vi "sposta nuove colonne.vi"(11 "Array 5":string[][](array[string])) -> (3 "Array 4":string[][](array[string]))   [LabVIEW 2019]
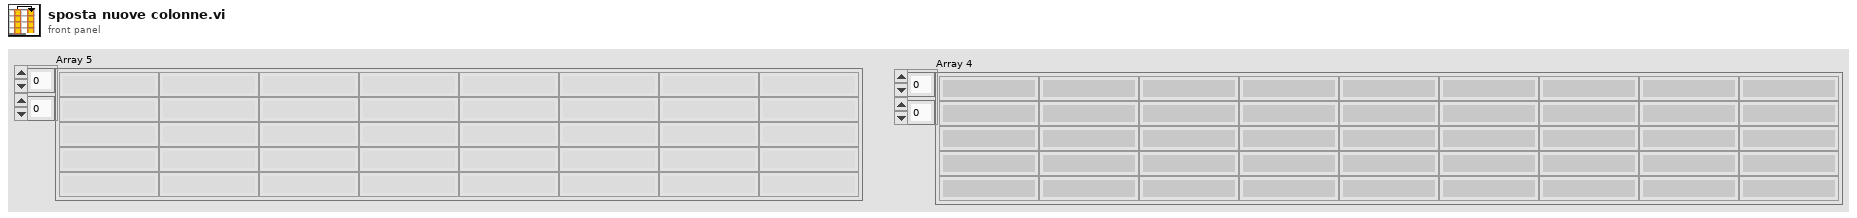
[diagram p1: front panel]
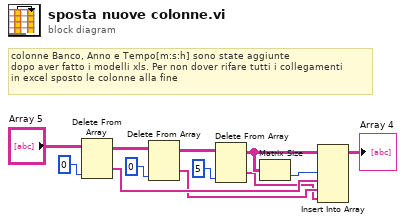
[diagram p0: block diagram]
diagram:
  # "colonne Banco, Anno e Tempo[m:s:h] sono state aggiunte\ndopo aver fatto i modelli xls. Per non dover rifare tutti i collegamenti\nin excel sposto le colonne alla fine"
  n1 = Delete From Array(array="Array 5", index (col)=0 ("disabled index (col)")) -> (deleted portion=w3:string[], array with subset deleted=w9:string[][])  [unwired: 2 in]
  n2 = Delete From Array(array=w9, index (col)=0 ("disabled index (col)")) -> (deleted portion=w2:string[], array with subset deleted=w11:string[][])  [unwired: 2 in]
  n3 = Delete From Array(array=w11, index (col)=5 ("disabled index (col)")) -> (deleted portion=w1:string[], array with subset deleted=w6:string[][])  [unwired: 2 in]
  n4 = Matrix Size(0:w6) -> (2:w5:i32)  [unwired: 1 out]
  n5 = Insert Into Array(array=w6, index (col)=w5, new element #1=w3, new element #2=w2, new element #3=w1) -> (→"Array 4":string[][])  [unwired: 1 in]
